vi "LogError_String.vi"(8 "error in (no error)":errorcluster, 9 "code(0)":i32, 10 "log string":string, 11 "qbus in":refnum<class "Qbus.lvclass">=refnum) -> (0 "error out":errorcluster, 3 "qbus out":refnum<class "Qbus.lvclass">)   [LabVIEW 2016, in "TraceLogger.lvlib"]
doc: "Logs a tracepoint instance that includes a custom error description and an error code."
uses:
  <vilib>/addons/TraceLogger/TraceLogger.lvlib
  <vilib>/addons/Qbus/Qbus.lvclass
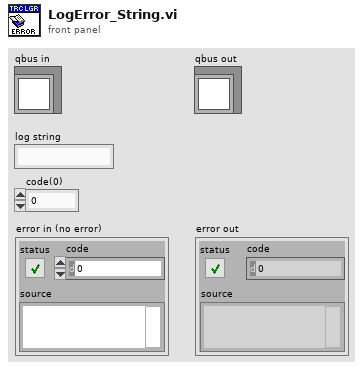
[diagram p1: front panel]
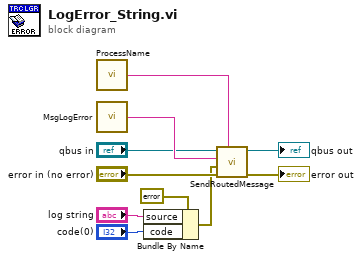
[diagram p0: block diagram]
diagram:
  n1 = call <vilib>:"ProcessName.vi"() -> ("process name"=w7:string)  [unwired: 5 in]
  n2 = call <vilib>:"MsgLogError.vi"() -> ("message name"=w9:string)  [unwired: 5 in]
  n3 = Bundle By Name(cluster=errorcluster {"status"=FALSE, "code"=0, "source"=""} ("error"), "source"="log string", "code"="code(0)") -> (w3:errorcluster)
  n4 = call <vilib>:"SendRoutedMessage.vi"("listener process"=w7, "error in (no error)"="error in (no error)", "message value"=w3, "message name"=w9, "Qbus in"="qbus in") -> ("error in (no error)"=→"error out":errorcluster, "Qbus out"=→"qbus out":refnum<class "Qbus.lvclass">)  [unwired: 5 in]
